vi "PathData.vi"() -> (0 "OhanaOS Path":path)   [LabVIEW 2009]
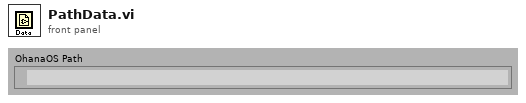
[diagram p1: front panel]
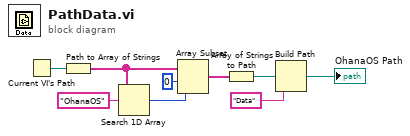
[diagram p0: block diagram]
diagram:
  n1 = Current VI's Path() -> (path=w9:path)
  n2 = Path to Array of Strings(0:w9) -> (2:w7:string[])  [unwired: 1 out]
  n3 = Search 1D Array(1D array=w7, element="OhanaOS" ("élément")) -> (index of element=w4:i32)  [unwired: 1 out]
  n4 = Array Subset(array=w7, index=0 ("Indice du tableau"), length=w4) -> (w5:string[])
  n5 = Array of Strings to Path(0:w5) -> (2:w3:path)  [unwired: 1 out]
  n6 = Build Path(base path=w3, name or relative path="Data" ("nom ou chemin relatif")) -> (appended path=→"OhanaOS Path":path)
